vi "Write basicType.vi"(10 "basicType":refnum<class "Primitive.lvclass">, 11 "Array in":refnum<class "Array.lvclass">) -> (3 "Array out":refnum<class "Array.lvclass">)   [LabVIEW 2013, in "Array.lvclass"]
uses:
  Array.lvclass
  Primitive/Primitive.lvclass
  Array.lvclass/Array.ctl
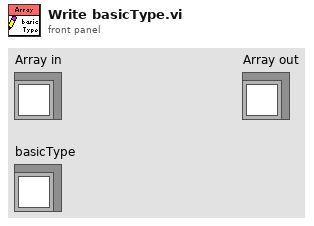
[diagram p1: front panel]
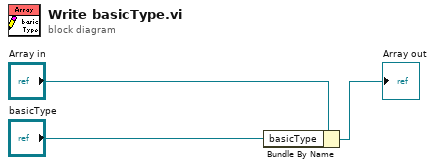
[diagram p0: block diagram]
diagram:
  n1 = Bundle By Name(cluster="Array in", "basicType"="basicType") -> (→"Array out":refnum<class "Array.lvclass">)
